vi "计算加标体积.vi"(8 "error in (no error)":errorcluster caption="错误输入（无错误）", 11 "参数":enum16{"氨氮", "总磷", "总氮", "CODMn", "CODcr"}(ring)) -> (0 "error out":errorcluster caption="错误输出", 2 "加标后理论浓度":dbl, 3 "加标体积":dbl)   [LabVIEW 2016, in "质控单元.lvlib"]
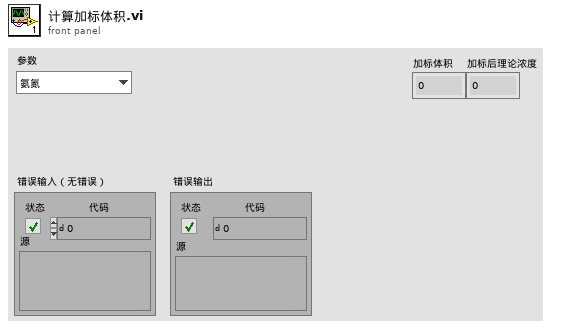
[diagram p1: front panel]
types:
  T1 = cluster{"因子编码":u32, "单位":u16, "标样参考值":sgl, "水样数据时间":timestamp, "水样实测值":sgl, "水样数据标识":string, "标样数据时间":timestamp, "标样实测值":sgl, "标样数据标识":string, "空白数据时间":timestamp, "空白实测值":sgl, "空白数据标识":string, "零点核查数据时间":timestamp, "零点核查实测值":sgl, "零点核查数据标识":string, "跨度核查数据时间":timestamp, "跨度核查实测值":sgl, "跨度核查数据标识":string, "加标回收数据时间":timestamp, "加标回收实测值":sgl, "加标回收数据标识":string, "平行样数据时间":timestamp, "平行样实测值":sgl, "平行样数据标识":string}
  T2 = cluster{"量程":dbl, "检出限":dbl, "加标前水样浓度":dbl, "加标后水样浓度":dbl, "加标水杯定容体积":dbl, "加标母液浓度":dbl, "加标体积":dbl, "加标回收率":dbl}
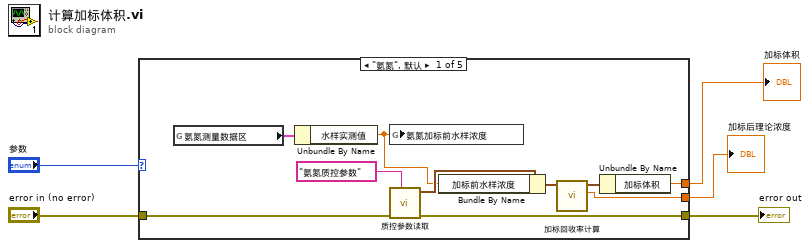
[diagram p0: block diagram]
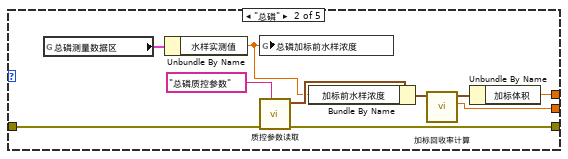
[diagram p2: hidden frame]
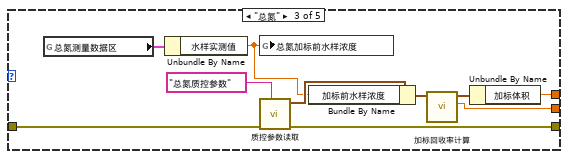
[diagram p3: hidden frame]
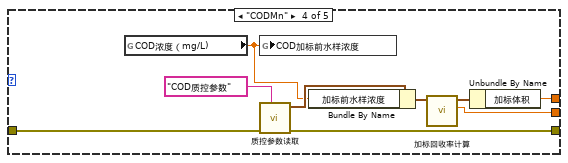
[diagram p4: hidden frame]
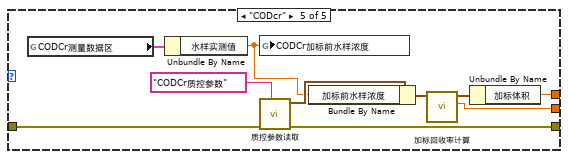
[diagram p5: hidden frame]
diagram:
  n1 = case shown="\"氨氮\", 默认" "参数" {
    tunnel: "error in (no error)" -> [w9 w16 w26 w36 w45]
    tunnel: [w8 w17 w27 w37 w46] -> w3
    tunnel: [w7 w18 w28 w38 w47] -> w1
    tunnel: [w6 w19 w29 w39 w48] -> w2
    frame "氨氮", Default {
      n2 = global read "与氨氮交互全局.vi" "氨氮测量数据区"() -> (w10:T1)
      n3 = Unbundle By Name(w10) -> ("水样实测值"=w11:sgl)
      n4 = global write "水样浓度全局.vi" "氨氮加标前水样浓度"(w11) -> ()
      n5 = call "质控参数读取.vi"("section"="氨氮质控参数", "error in (no error)"=w9) -> ("error out"=w8:errorcluster, "参数"=w13:T2)  [unwired: 8 in]
      n6 = Bundle By Name(cluster=w13, "加标前水样浓度"=w11) -> (w14:T2)
      n7 = call "加标回收率计算.vi"("参数"=w14) -> ("加标后理论浓度"=w7:dbl, "参数 out"=w12:T2)  [unwired: 9 in]
      n8 = Unbundle By Name(w12) -> ("加标体积"=w6:dbl)
    }
    frame "总磷" {
      n9 = global read "与总磷交互全局.vi" "总磷测量数据区"() -> (w21:T1)
      n10 = Unbundle By Name(w21) -> ("水样实测值"=w20:sgl)
      n11 = global write "水样浓度全局.vi" "总磷加标前水样浓度"(w20) -> ()
      n12 = call "质控参数读取.vi"("section"="总磷质控参数", "error in (no error)"=w16) -> ("error out"=w17:errorcluster, "参数"=w22:T2)  [unwired: 8 in]
      n13 = Bundle By Name(cluster=w22, "加标前水样浓度"=w20) -> (w24:T2)
      n14 = call "加标回收率计算.vi"("参数"=w24) -> ("加标后理论浓度"=w18:dbl, "参数 out"=w23:T2)  [unwired: 9 in]
      n15 = Unbundle By Name(w23) -> ("加标体积"=w19:dbl)
    }
    frame "总氮" {
      n16 = global read "与总氮交互全局.vi" "总氮测量数据区"() -> (w30:T1)
      n17 = Unbundle By Name(w30) -> ("水样实测值"=w31:sgl)
      n18 = global write "水样浓度全局.vi" "总氮加标前水样浓度"(w31) -> ()
      n19 = call "质控参数读取.vi"("section"="总氮质控参数", "error in (no error)"=w26) -> ("error out"=w27:errorcluster, "参数"=w32:T2)  [unwired: 8 in]
      n20 = Bundle By Name(cluster=w32, "加标前水样浓度"=w31) -> (w34:T2)
      n21 = call "加标回收率计算.vi"("参数"=w34) -> ("加标后理论浓度"=w28:dbl, "参数 out"=w33:T2)  [unwired: 9 in]
      n22 = Unbundle By Name(w33) -> ("加标体积"=w29:dbl)
    }
    frame "CODMn" {
      n23 = global read "与CODMn交互全局.vi" "COD浓度（mg/L)"() -> (w40:dbl)
      n24 = global write "水样浓度全局.vi" "COD加标前水样浓度"(w40) -> ()
      n25 = call "质控参数读取.vi"("section"="COD质控参数", "error in (no error)"=w36) -> ("error out"=w37:errorcluster, "参数"=w42:T2)  [unwired: 8 in]
      n26 = Bundle By Name(cluster=w42, "加标前水样浓度"=w40) -> (w43:T2)
      n27 = call "加标回收率计算.vi"("参数"=w43) -> ("加标后理论浓度"=w38:dbl, "参数 out"=w41:T2)  [unwired: 9 in]
      n28 = Unbundle By Name(w41) -> ("加标体积"=w39:dbl)
    }
    frame "CODcr" {
      n29 = global read "与CODCr交互全局.vi" "CODCr测量数据区"() -> (w49:T1)
      n30 = Unbundle By Name(w49) -> ("水样实测值"=w50:sgl)
      n31 = global write "水样浓度全局.vi" "CODCr加标前水样浓度"(w50) -> ()
      n32 = call "质控参数读取.vi"("section"="CODCr质控参数", "error in (no error)"=w45) -> ("error out"=w46:errorcluster, "参数"=w52:T2)  [unwired: 8 in]
      n33 = Bundle By Name(cluster=w52, "加标前水样浓度"=w50) -> (w53:T2)
      n34 = call "加标回收率计算.vi"("参数"=w53) -> ("加标后理论浓度"=w47:dbl, "参数 out"=w51:T2)  [unwired: 9 in]
      n35 = Unbundle By Name(w51) -> ("加标体积"=w48:dbl)
    }
  }
  "error out" <- w3
  "加标体积" <- w2
  "加标后理论浓度" <- w1
